vi "Ex2Task1_Main.vi"() -> ()   [LabVIEW 2014, in "Ex2Task1.lvrbt"]
uses:
  Ex2Task1.lvrbt
  <vilib>/NXT/Dual Mode Library/Display/drawText.vi
panel:
  out "Result":dbl
  out "A+B":dbl
  in  "B":dbl
  in  "A":dbl
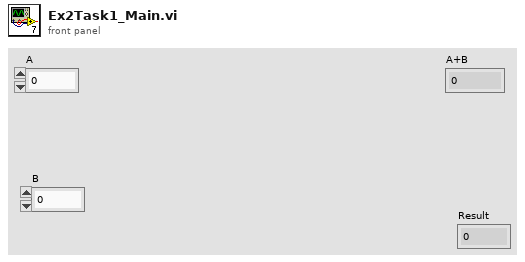
[diagram p1: front panel]
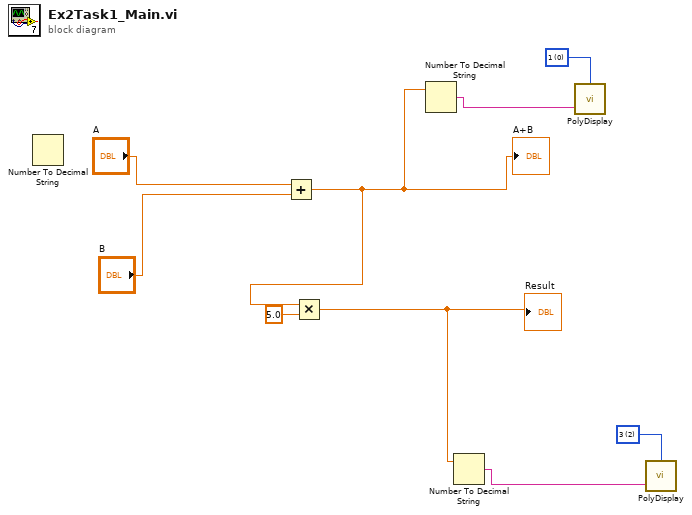
[diagram p0: block diagram]
diagram:
  w1 = i16 2 items=["1", "2", "3", "4", "5", "6", "7", "8", "9", "10", "11", "12"] ("Line")
  w4 = i16 0 items=["1", "2", "3", "4", "5", "6", "7", "8", "9", "10", "11", "12"] ("Line")
  n1 = Number To Decimal String() -> ()  [unwired: 2 in, 1 out]
  n2 = Add(x="A", y="B") -> (x+y=w6:dbl)
  "A+B" <- w6
  n3 = Multiply(x=w6, y=5.0) -> (x*y=w3:dbl)
  "Result" <- w3
  n4 = Number To Decimal String(number=w6) -> (decimal integer string=w5:string)  [unwired: 1 in]
  n5 = Number To Decimal String(number=w3) -> (decimal integer string=w2:string)  [unwired: 1 in]
  n6 = call-poly <vilib>:"PolyDisplay.vi"("Text"=w5, "Line"=w4) -> ()  [unwired: 2 in, 1 out]
  n7 = call-poly <vilib>:"PolyDisplay.vi"("Text"=w2, "Line"=w1) -> ()  [unwired: 2 in, 1 out]
